vi "ConnectToRobot.vi"(0 "error in":errorcluster, 1 "address":string, 2 "Telnet enable":bool, 3 "Telnet KCL password":string, 4 "SNPX enable":bool, 5 "FTP enable":bool, 6 "FTP user":string, 7 "FTP password":string) -> (20 "error out":errorcluster, 21 "robot":refnum<k24>, 24 "Telnet":refnum<k24>, 25 "Ftp":refnum<k24>, 26 "Snpx":refnum<k24>)   [LabVIEW 2016, in "UnderAutomation.Fanuc.lvlib"]
uses:
  UnderAutomation.Fanuc.lvlib
  C:/Users/fg/Documents/Fanuc.vi/LabVIEW_2024/UnderAutomation.Fanuc/lib/UnderAutomation.Fanuc.dll
  LabVIEW_2024/UnderAutomation.Fanuc/lib/UnderAutomation.Fanuc.dll
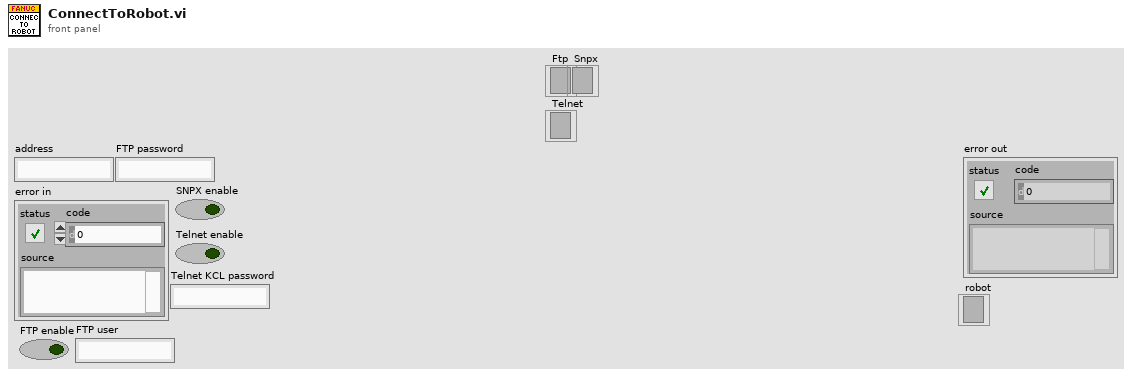
[diagram p1: front panel]
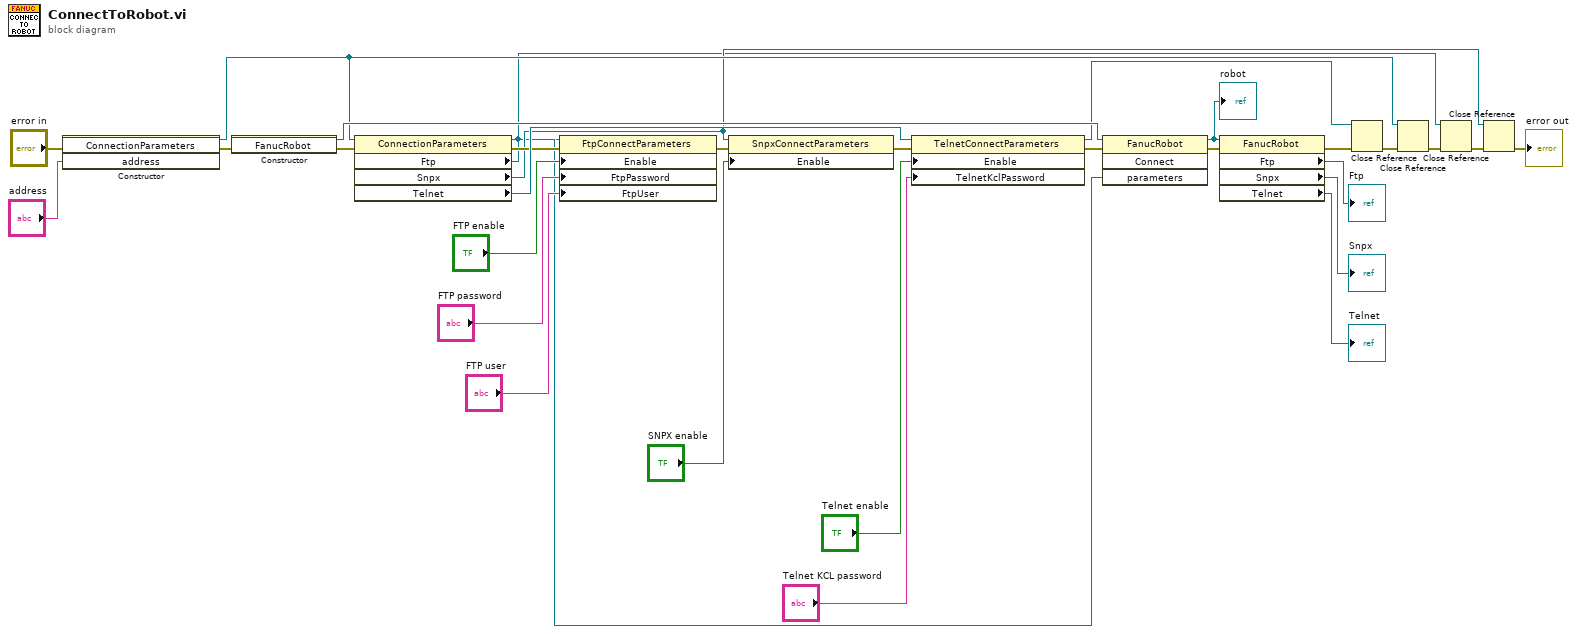
[diagram p0: block diagram]
diagram:
  n1 = constructor class="ConnectionParameters"(error in="error in", "address"="address") -> (reference out=w7:refnum<k24>, error out=w30:errorcluster)  [unwired: 2 in, 2 out]
  n2 = constructor class="FanucRobot"(error in=w30) -> (reference out=w31:refnum<k24>, error out=w23:errorcluster)  [unwired: 2 in, 1 out]
  n3 = property class="ConnectionParameters"(reference=w7, error in=w23) -> (reference out=w5:refnum<k24>, error out=w26:errorcluster, "Ftp"=w4:refnum<k24>, "Snpx"=w6:refnum<k24>, "Telnet"=w28:refnum<k24>)
  n4 = property class="FtpConnectParameters"(reference=w4, error in=w26, "Enable"="FTP enable", "FtpPassword"="FTP password", "FtpUser"="FTP user") -> (error out=w25:errorcluster)  [unwired: 1 out]
  n5 = property class="SnpxConnectParameters"(reference=w6, error in=w25, "Enable"="SNPX enable") -> (error out=w24:errorcluster)  [unwired: 1 out]
  n6 = property class="TelnetConnectParameters"(reference=w28, error in=w24, "Enable"="Telnet enable", "TelnetKclPassword"="Telnet KCL password") -> (reference out=w10:refnum<k24>, error out=w22:errorcluster)
  n7 = invoke class="FanucRobot" method="Connect"(reference=w31, error in=w22, "parameters"=w5) -> (reference out=w15:refnum<k24>, error out=w14:errorcluster)  [unwired: 1 in, 2 out]
  "robot" <- w15
  n8 = property class="FanucRobot"(reference=w15, error in=w14) -> (error out=w9:errorcluster, "Ftp"=→"Ftp":refnum<k24>, "Snpx"=→"Snpx":refnum<k24>, "Telnet"=→"Telnet":refnum<k24>)  [unwired: 1 out]
  n9 = Close Reference(reference=w10, error in (no error)=w9) -> (error out=w8:errorcluster)
  n10 = Close Reference(reference=w7, error in (no error)=w8) -> (error out=w3:errorcluster)
  n11 = Close Reference(reference=w4, error in (no error)=w3) -> (error out=w2:errorcluster)
  n12 = Close Reference(reference=w6, error in (no error)=w2) -> (error out=→"error out":errorcluster)
